vi "Drive Motor Recieve.vi"(10 "Drive Motor Handle In":T1, 11 "Error In":errorcluster) -> (2 "Drive Motor Handle Out":T1, 3 "Error Out":errorcluster)   [LabVIEW 2019]
uses:
  Drive Motor Handle.ctl
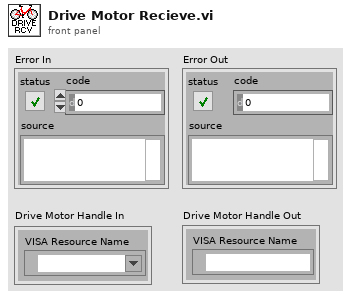
[diagram p1: front panel]
types:
  T1 = typedef "Drive Motor Handle.ctl" = cluster{"VISA Resource Name":refnum<visa-resource-name>}
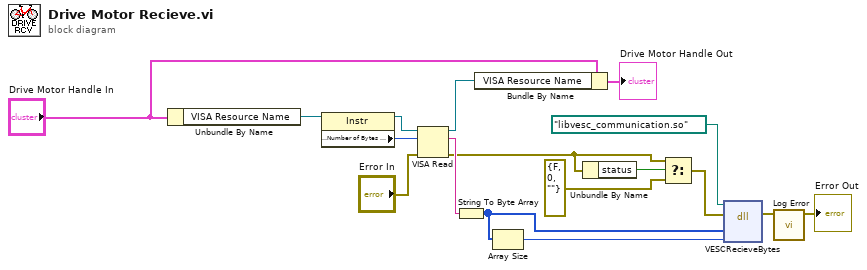
[diagram p0: block diagram]
diagram:
  n1 = Unbundle By Name("Drive Motor Handle In") -> ("VISA Resource Name"=w9:refnum<visa-resource-name>)
  n2 = property class="Instr"(reference=w9) -> (reference out=w1:refnum<visa-resource-name>, "Serial Settings:Number of Bytes at Serial Port"=w8:u32)  [unwired: 1 in, 1 out]
  n3 = VISA Read(VISA resource name=w1, byte count=w8, error in (no error)="Error In") -> (VISA resource name out=w3:refnum<visa-resource-name>, read buffer=w6:string, error out=w5:errorcluster)  [unwired: 1 out]
  n4 = String To Byte Array(string=w6) -> (unsigned byte array=w16:u8[])
  n5 = Bundle By Name(cluster="Drive Motor Handle In", "VISA Resource Name"=w3) -> (→"Drive Motor Handle Out":T1)
  n6 = Array Size(array=w16) -> (size(s)=w17:i32)
  n7 = Unbundle By Name(w5) -> ("status"=w12:bool)
  n8 = Select(t=w5, s=w12, f=errorcluster {"status"=FALSE, "code"=0, "source"=""}) -> (s? t:f=w11:errorcluster)
  n9 = dll-call lib="?" fn="VESCRecieveBytes"(path in=path "libvesc_communication.so", error in=w11, "bytes"=w16, "length"=w17) -> (error out=w14:errorcluster)  [unwired: 4 in, 1 out]
  n10 = call "Log Error.vi"("Error In"=w14) -> ("Error Out"=→"Error Out":errorcluster)  [unwired: 10 in]
